vi "Move.vi"(7 "Wall Positions":T1[](array[typedef]), 8 "error in (no error)":errorcluster, 9 "GameBoard Size":T1, 10 "Move":T2, 11 "object in":refnum<class "Piece of Bricks.lvclass">) -> (0 "error out":errorcluster, 2 "Freeze Piece":bool, 3 "object out":refnum<class "Piece of Bricks.lvclass">)   [LabVIEW 2017, in "Piece of Bricks.lvclass"]
uses:
  Piece of Bricks.lvclass
  Controls/Moves.ctl
  Controls/Coordinates.ctl
  Piece of Bricks.lvclass/Piece of Bricks.ctl
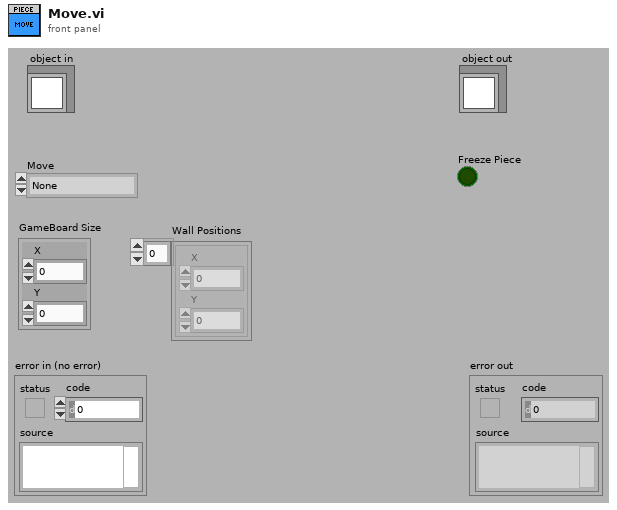
[diagram p1: front panel]
types:
  T1 = typedef "Coordinates.ctl" = cluster{"X":i32, "Y":i32}
  T2 = typedef "Moves.ctl" = enum16{"None", "Right", "Left", "Step Down", "Go Down", "90 Clockwise", "90 Anti-Clockwise"}
  T3 = typedef "Piece Description.ctl" = cluster{"Pieces Geometry Names":T4, "Piece Color":u32, "Coordinates":T1[], "X Offset":i32, "Y Offset":i32, "Rotation State":T5}
  T4 = typedef "Pieces Geometry Names.ctl" = enum16{"I", "O", "T", "L", "J", "Z", "S"}
  T5 = typedef "Rotation State.ctl" = enum16{"0", "90", "180", "270"}
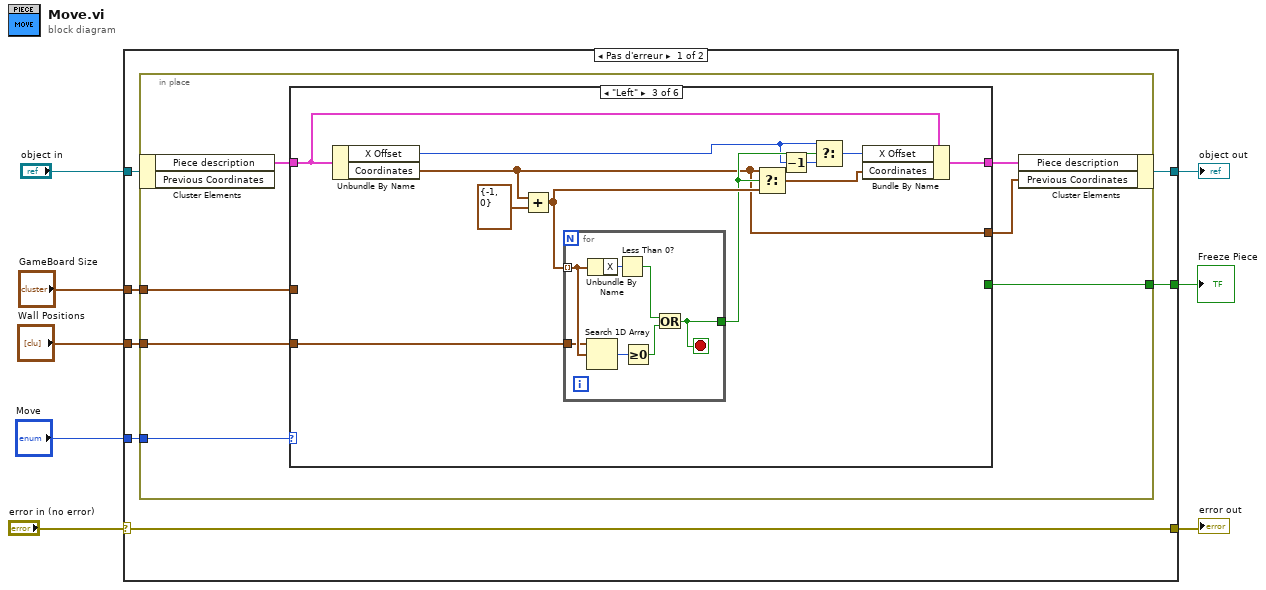
[diagram p0: block diagram]
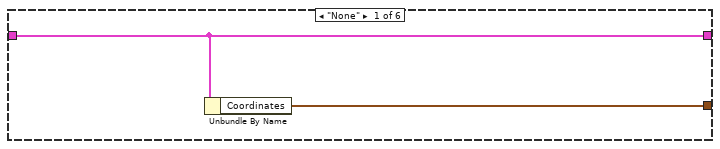
[diagram p2: hidden frame]
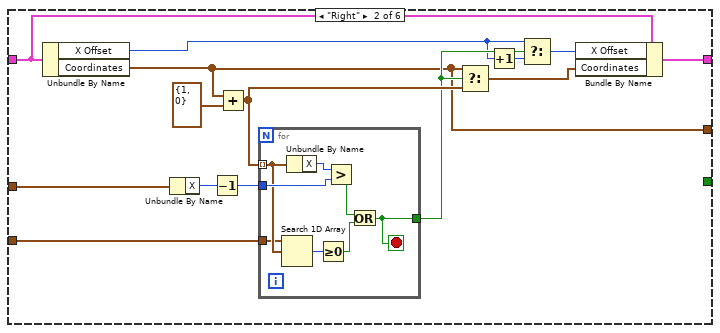
[diagram p3: hidden frame]
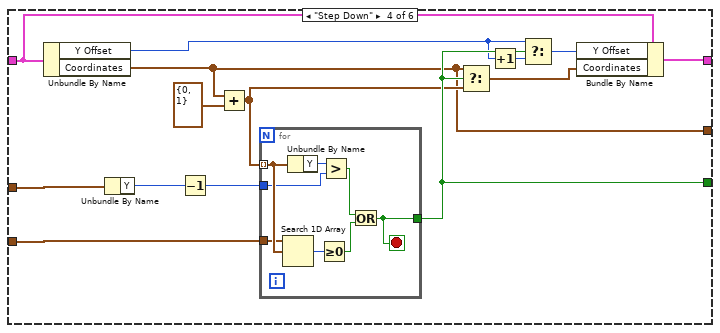
[diagram p4: hidden frame]
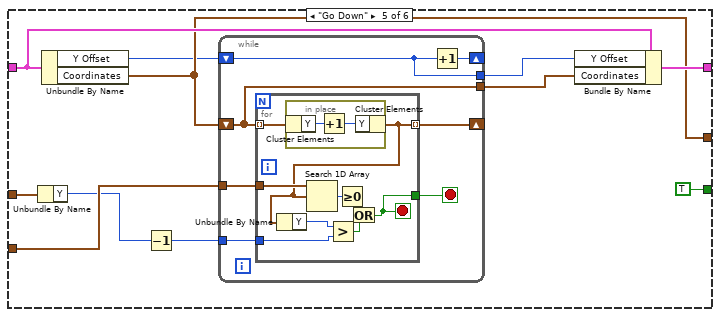
[diagram p5: hidden frame]
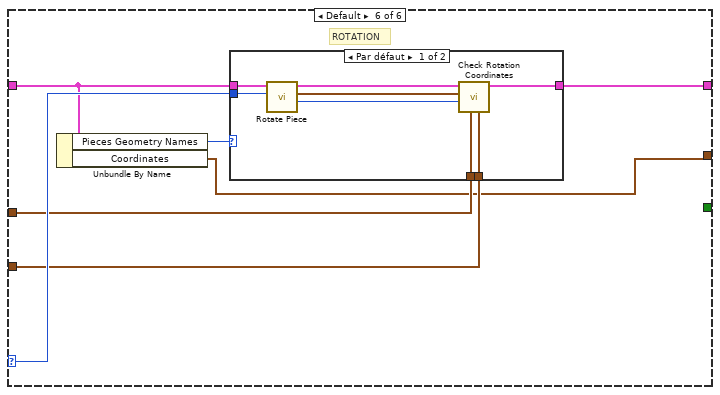
[diagram p6: hidden frame]
diagram:
  n1 = case shown="Pas d'erreur" "error in (no error)" {
    selector: "error in (no error)" -> [w10 w133]
    tunnel: [w10 w133] -> w7
    tunnel: [w14 w132] -> w2
    tunnel: "object in" -> [w15 w132]
    tunnel: "Move" -> [w13 _]
    tunnel: "GameBoard Size" -> [w12 _]
    tunnel: "Wall Positions" -> [w11 _]
    tunnel: [w9 _] -> w1
    frame No Error {
      n2 = in-place {
        in-place-border: w13 -> [w22]
        in-place-border: w12 -> [w19]
        in-place-border: w11 -> [w18]
        in-place-border: [w17] -> w9
        n3 = in-place-cluster #1(w15) -> ("Piece description"=w21:T3)  [unwired: 1 out]
        n4 = case shown="\"Left\"" w22 {
          selector: w22 -> [_ _ _ _ _ w122]
          tunnel: w21 -> [w24 w36 w56 w78 w97 w118]
          tunnel: [w24 w35 w55 w77 w96 w121] -> w20
          tunnel: w19 -> [_ w38 _ w76 w95 w120]
          tunnel: w18 -> [_ w37 w57 w75 w94 w119]
          tunnel: [_ _ _ w74 TRUE _] -> w17
          tunnel: [w23 w25 w47 w65 w92 w116] -> w16
          frame "None" {
            n5 = Unbundle By Name(w24) -> ("Coordinates"=w23:T1[])
          }
          frame "Right" {
            n6 = Unbundle By Name(w36) -> ("X Offset"=w28:i32, "Coordinates"=w25:T1[])
            n7 = Unbundle By Name(w38) -> ("X"=w33:i32)
            n8 = Decrement(x=w33) -> (x-1=w26:i32)
            n9 = Add(x=w25, y=T1 {"X"=1, "Y"=0} ("Coordinates")) -> (x+y=w32:T1[])
            n10 = for {
              tunnel: w26 -> [w45]
              tunnel: w32 -> [w43] mode=indexing
              tunnel: w37 -> [w42]
              tunnel: [w39] -> w29
              stop <- w39 stop-if-true
              n11 = Search 1D Array(1D array=w42, element=w43) -> (index of element=w44:i32)  [unwired: 1 in]
              n12 = Unbundle By Name(w43) -> ("X"=w46:i32)
              n13 = Greater Or Equal To 0?(x=w44) -> (x >= 0?=w40:bool)
              n14 = Greater?(x=w46, y=w45) -> (0:w41:bool)
              n15 = Or(x=w41, y=w40) -> (x .or. y?=w39:bool)
            }
            n16 = Select(t=w25, s=w29, f=w32) -> (s? t:f=w31:T1[])
            n17 = Increment(x=w28) -> (x+1=w27:i32)
            n18 = Select(t=w28, s=w29, f=w27) -> (s? t:f=w30:i32)
            n19 = Bundle By Name(cluster=w36, "X Offset"=w30, "Coordinates"=w31) -> (w35:T3)
          }
          frame "Left" {
            n20 = Unbundle By Name(w56) -> ("X Offset"=w48:i32, "Coordinates"=w47:T1[])
            n21 = Add(x=w47, y=T1 {"X"=-1, "Y"=0} ("Coordinates")) -> (x+y=w53:T1[])
            n22 = for {
              tunnel: w53 -> [w62] mode=indexing
              tunnel: w57 -> [w61]
              tunnel: [w58] -> w50
              stop <- w58 stop-if-true
              n23 = Search 1D Array(1D array=w61, element=w62) -> (index of element=w63:i32)  [unwired: 1 in]
              n24 = Unbundle By Name(w62) -> ("X"=w64:i32)
              n25 = Less Than 0?(x=w64) -> (x < 0?=w60:bool)
              n26 = Greater Or Equal To 0?(x=w63) -> (x >= 0?=w59:bool)
              n27 = Or(x=w60, y=w59) -> (x .or. y?=w58:bool)
            }
            n28 = Select(t=w47, s=w50, f=w53) -> (s? t:f=w52:T1[])
            n29 = Decrement(x=w48) -> (x-1=w49:i32)
            n30 = Select(t=w48, s=w50, f=w49) -> (s? t:f=w51:i32)
            n31 = Bundle By Name(cluster=w56, "X Offset"=w51, "Coordinates"=w52) -> (w55:T3)
          }
          frame "Step Down" {
            n32 = Unbundle By Name(w78) -> ("Y Offset"=w69:i32, "Coordinates"=w65:T1[])
            n33 = Unbundle By Name(w76) -> ("Y"=w67:i32)
            n34 = Decrement(x=w67) -> (x-1=w66:i32)
            n35 = Add(x=w65, y=T1 {"X"=0, "Y"=1} ("Coordinates")) -> (x+y=w72:T1[])
            n36 = for {
              tunnel: w72 -> [w84] mode=indexing
              tunnel: w75 -> [w83]
              tunnel: [w80] -> w74
              tunnel: w66 -> [w79]
              stop <- w80 stop-if-true
              n37 = Search 1D Array(1D array=w83, element=w84) -> (index of element=w85:i32)  [unwired: 1 in]
              n38 = Unbundle By Name(w84) -> ("Y"=w86:i32)
              n39 = Greater Or Equal To 0?(x=w85) -> (x >= 0?=w81:bool)
              n40 = Greater?(x=w86, y=w79) -> (0:w82:bool)
              n41 = Or(x=w82, y=w81) -> (x .or. y?=w80:bool)
            }
            n42 = Select(t=w65, s=w74, f=w72) -> (s? t:f=w71:T1[])
            n43 = Increment(x=w69) -> (x+1=w68:i32)
            n44 = Select(t=w69, s=w74, f=w68) -> (s? t:f=w70:i32)
            n45 = Bundle By Name(cluster=w78, "Y Offset"=w70, "Coordinates"=w71) -> (w77:T3)
          }
          frame "Go Down" {
            n46 = Unbundle By Name(w95) -> ("Y"=w90:i32)
            n47 = Unbundle By Name(w97) -> ("Y Offset"=w91:i32, "Coordinates"=w92:T1[])
            n48 = Decrement(x=w90) -> (x-1=w89:i32)
            n49 = while {
              tunnel: w94 -> [w104]
              tunnel: w89 -> [w102]
              shift-right: [w101] -> _
              shift-left: w92 -> [w98]
              shift-right: [w100] -> _
              shift-left: w91 -> [w99]
              tunnel: [w99] -> w88
              tunnel: [w98] -> w87
              stop <- w103 stop-if-true
              n50 = for {
                tunnel: w98 -> [w113] mode=indexing
                tunnel: w104 -> [w112]
                tunnel: [w105] -> w103
                tunnel: [w110] -> w101 mode=indexing
                tunnel: w102 -> [w108]
                stop <- w105 stop-if-true
                n51 = in-place {
                  n52 = in-place-cluster #2(w113) -> ("Y"=w115:i32)
                  n53 = Increment(x=w115) -> (x+1=w114:i32)
                  n54 = in-place-cluster #2("Y"=w114) -> (w110:T1)
                }
                n55 = Unbundle By Name(w110) -> ("Y"=w109:i32)
                n56 = Search 1D Array(1D array=w112, element=w110) -> (index of element=w111:i32)  [unwired: 1 in]
                n57 = Greater?(x=w109, y=w108) -> (0:w107:bool)
                n58 = Greater Or Equal To 0?(x=w111) -> (x >= 0?=w106:bool)
                n59 = Or(x=w106, y=w107) -> (x .or. y?=w105:bool)
              }
              n60 = Increment(x=w99) -> (x+1=w100:i32)
            }
            n61 = Bundle By Name(cluster=w97, "Y Offset"=w88, "Coordinates"=w87) -> (w96:T3)
          }
          frame Default {
            # "ROTATION"
            n62 = Unbundle By Name(w118) -> ("Pieces Geometry Names"=w117:T4, "Coordinates"=w116:T1[])
            n63 = case shown="Par défaut" w117 {
              tunnel: w122 -> [w130 _]
              tunnel: [w129 w131] -> w121
              tunnel: w120 -> [w127 _]
              tunnel: w118 -> [w126 w131]
              tunnel: w119 -> [w124 _]
              frame Default {
                n64 = call "Rotate Piece.vi"("Move"=w130, "Piece Description"=w126) -> ("New Rotation State"=w123:T5, "Rotated Coordinates"=w128:T1[], "Piece Description Out"=w125:T3)  [unwired: 6 in, 1 out]
                n65 = call "Check Rotation Coordinates.vi"("Wall Positions"=w124, "GameBoard Size"=w127, "New Rotation State"=w123, "Rotated Coordinates"=w128, "Piece description"=w125) -> ("Piece description Out"=w129:T3)  [unwired: 5 in, 1 out]
              }
              frame "O" {
              }
            }
          }
        }
        n66 = in-place-cluster #1("Piece description"=w20, "Previous Coordinates"=w16) -> (w14:refnum<class "Piece of Bricks.lvclass">)
      }
    }
    frame Error {
    }
  }
  "error out" <- w7
  "object out" <- w2
  "Freeze Piece" <- w1
